vi "SCAN_VISA.vi"(8 "entrée d'erreur (pas d'erreur)":errorcluster) -> (0 "sortie d'erreur":errorcluster, 3 "Refnum VISA en sortie":refnum<visa-resource-name>)   [LabVIEW 2020]
uses:
  <vilib>/Instr/_visa.llb/VISA Find Search Mode.ctl
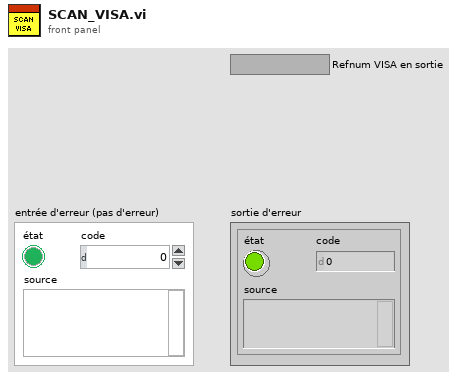
[diagram p1: front panel]
types:
  T1 = typedef "VISA Find Search Mode.ctl" = u32
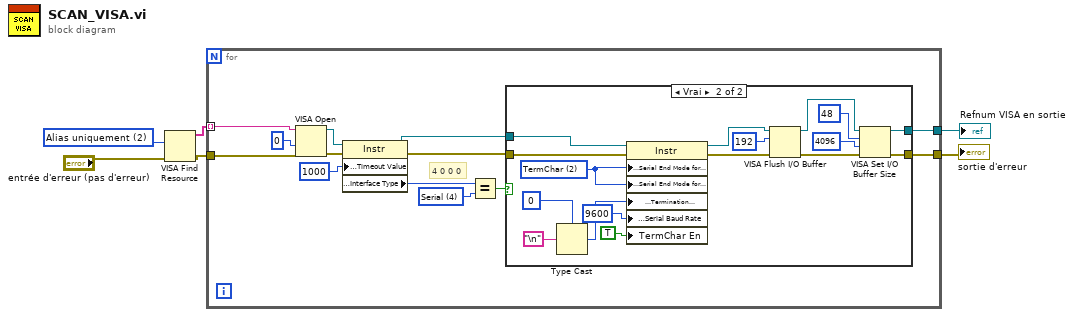
[diagram p0: block diagram]
diagram:
  w1 = T1 2 items=["Noms canoniques uniquement"=0, "Alias uniquement"=2, "Inclure les alias correspondants"=3, "Inclure tous les alias"=4] ("Search Mode")
  n1 = VISA Find Resource(8:"entrée d'erreur (pas d'erreur)", 10:w1) -> (0:w4:errorcluster, 3:w3:string[])  [unwired: 1 in, 1 out]
  n2 = for {
    tunnel: w3 -> [w10] mode=indexing
    tunnel: w4 -> [w9]
    tunnel: [w8] -> w5
    tunnel: [w7] -> w6
    w15 = u16 4 items=["GPIB"=1, "VXI"=2, "GPIB-VXI"=3, "Serial"=4, "PXI"=5, "TCPIP"=6, "USB"=7] ("Interface Information:Interface Type")
    # "4 0 0 0"
    n3 = VISA Open(access mode=u32 0, error in (no error)=w9, VISA resource name=w10) -> (VISA resource name=w17:refnum<visa-resource-name>, error out=w16:errorcluster)  [unwired: 2 in]
    n4 = property class="Instr"(reference=w17, error in=w16, "General Settings:Timeout Value"=u32 1000) -> (reference out=w12:refnum<visa-resource-name>, error out=w11:errorcluster, "Interface Information:Interface Type"=w14:u16)
    n5 = Equal?(x=w14, y=w15) -> (x = y?=w13:bool)
    n6 = case shown="Vrai" w13 {
      tunnel: [w20 w22] -> w8
      tunnel: [w21 w23] -> w7
      tunnel: w12 -> [w20 w37]
      tunnel: w11 -> [w21 w38]
      frame False {
        # "EDIT: Remove interfaces not supported by your instrument."
        # "GPIB, TCP/IP, and USB Interface"
      }
      frame True {
        w27 = u16 2 items=["None", "LastBit", "TermChar"] ("Serial Settings:Serial End Mode for Reads")
        n7 = Type Cast(type=u8 0, x="\n" ("Line Feed Constant")) -> (*(type *) &x=w26:u8)
        n8 = property class="Instr"(reference=w37, error in=w38, "Serial Settings:Serial End Mode for Reads"=w27, "Serial Settings:Serial End Mode for Writes"=w27, "Message Based Settings:Termination Character"=w26, "Serial Settings:Serial Baud Rate"=u32 9600 ("Serial Settings:Baud Rate"), "TermChar En"=TRUE ("Message Based Settings:Termination Character Enable")) -> (reference out=w33:refnum<visa-resource-name>, error out=w35:errorcluster)
        n9 = VISA Flush I/O Buffer(VISA resource name=w33, mask (16)=u16 192, error in (no error)=w35) -> (VISA resource name out=w36:refnum<visa-resource-name>, error out=w34:errorcluster)
        n10 = VISA Set I/O Buffer Size(VISA resource name=w36, mask (16)=u16 48, size (4096)=u32 4096 ("size (0)"), error in (no error)=w34) -> (VISA resource name out=w22:refnum<visa-resource-name>, error out=w23:errorcluster)
      }
    }
  }
  "Refnum VISA en sortie" <- w5
  "sortie d'erreur" <- w6
